vi "Main IU.vi"() -> ()   [LabVIEW 2018]
uses:
  <vilib>/Analysis/baseanly.llb/Mean (DBL).vi
  <vilib>/Analysis/NI_AALBase.lvlib
panel:
  out "Motor2":waveform(dbl)[](graph)
  out "Motor2":cluster{dbl, dbl, dbl}(graph)
  in  "Setpoint 2":dbl min=0.0 max=1.0 step=0.1
  out "rad/s":dbl(graph)
  out "Saving Data":bool
  in  "Record Button":bool
  in  "Filename":path=path "test.lvm"
  out "Motor1":waveform(dbl)[](graph)
  in  "Stop UI and RT":bool
  in  "Stop UI":bool
  in  "Setpoint1":dbl min=0.0 max=1.0 step=0.1
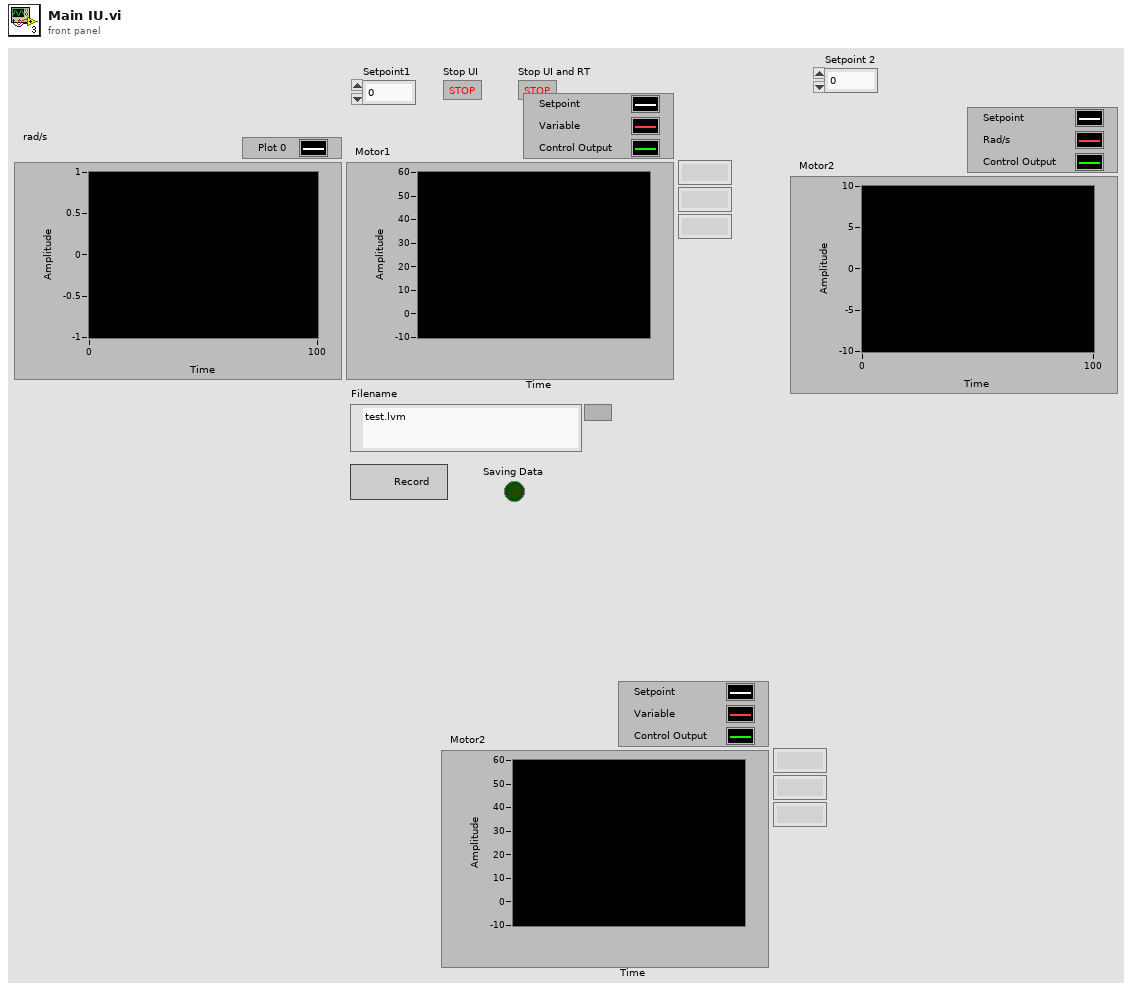
[diagram p1: front panel]
types:
  T1 = cluster{"Double":dbl, "dbl Scaled Value":dbl, "Output":dbl, "seconds since 1Jan1904":timestamp, dbl, dbl, dbl}
  T2 = cluster{"writer name":string, "Variant":variant, "Variant":variant}
  T3 = cluster{"Double":dbl, "dbl Scaled Value":dbl, "Output":dbl, "seconds since 1Jan1904":timestamp, dbl, dbl, dbl}[]
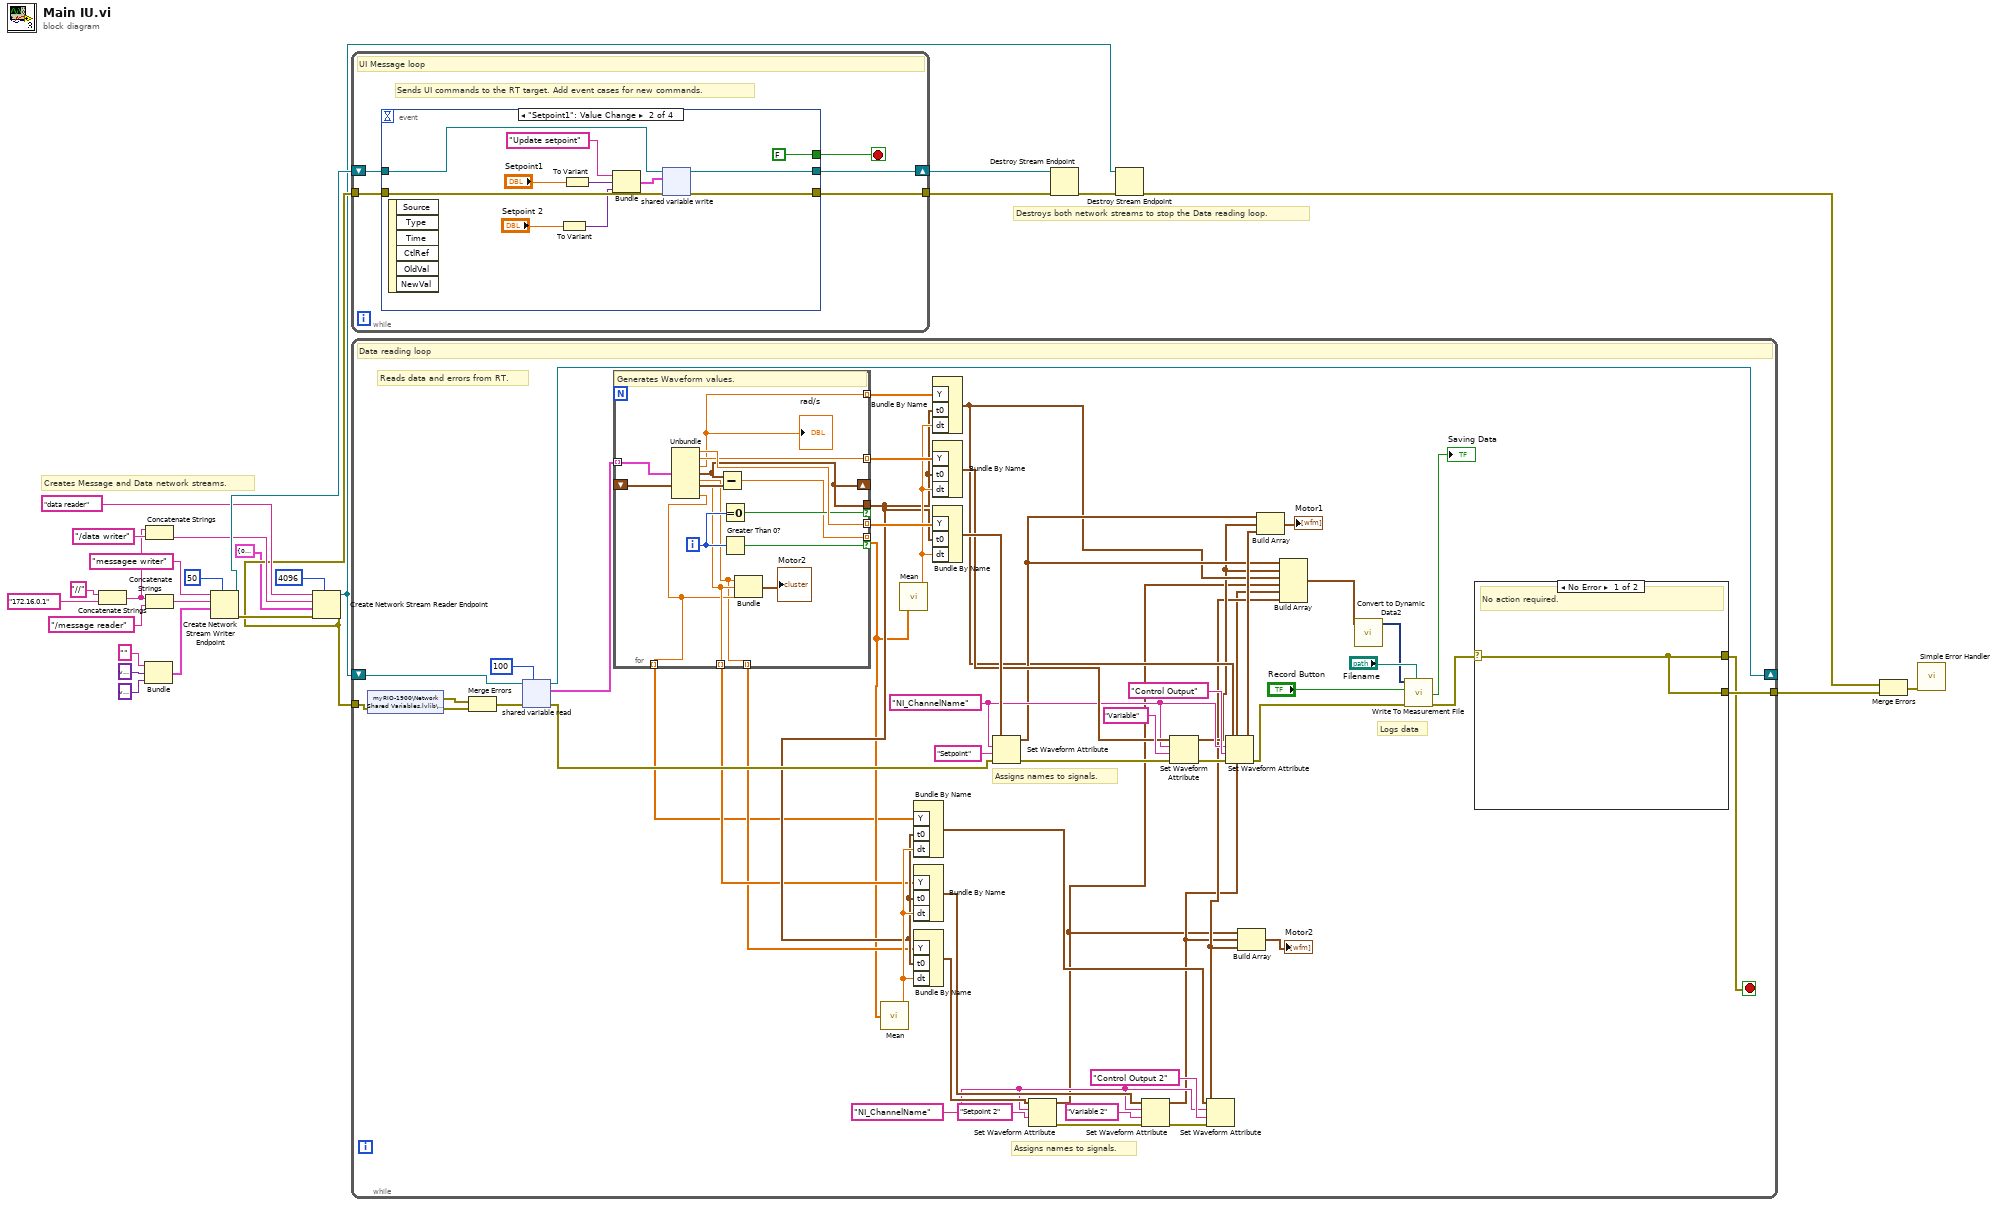
[diagram p0: block diagram]
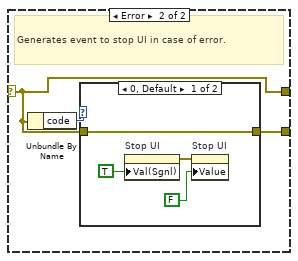
[diagram p2: hidden frame]
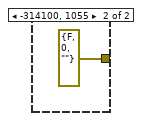
[diagram p3: hidden frame]
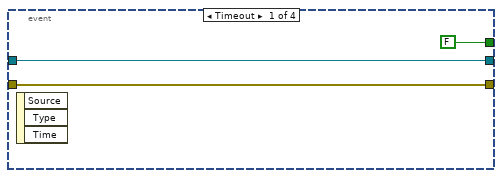
[diagram p4: hidden frame]
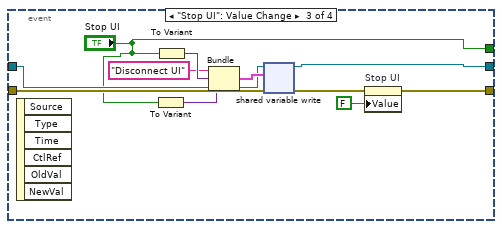
[diagram p5: hidden frame]
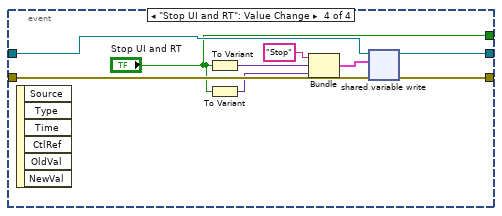
[diagram p6: hidden frame]
diagram:
  # "Destroys both network streams to stop the Data reading loop."
  # "Creates Message and Data network streams."
  n1 = Concatenate Strings("//", "172.16.0.1" ("myRIO IP")) -> (w2:string)
  n2 = Bundle("", variant, variant) -> (w26:cluster{string, variant, variant})  [unwired: 1 in]
  n3 = Concatenate Strings(w2, "/data writer") -> (w17:string)
  n4 = Concatenate Strings(w2, "/message reader") -> (w3:string)
  n5 = Create Network Stream Writer Endpoint(7:50 ("writer buffer size"), 9:w26, 10:w3, 11:"messagee writer" ("writer name")) -> (0:w14:errorcluster, 3:w20:refnum<k21>)  [unwired: 3 in]
  n6 = Create Network Stream Reader Endpoint(7:4096 ("reader buffer size"), 8:w14, 9:T1 {"Double"=0.0, "dbl Scaled Value"=0.0, "Output"=0.0, "seconds since 1Jan1904"=timestamp(0 s since 1904-01-01), 0.0, 0.0, 0.0} ("Data"), 10:w17, 11:"data reader" ("reader name")) -> (0:w13:errorcluster, 3:w6:refnum<k21>)  [unwired: 2 in]
  n7 = while {
    tunnel: w13 -> [w30]
    shift-right: [w29] -> w8
    shift-left: w20 -> [w31]
    tunnel: [w28] -> w9
    stop <- w27 stop-if-true
    # "Sends UI commands to the RT target. Add event cases for new commands."
    # "UI Message loop"
    n8 = event shown="[1] \"Setpoint1\": Value Change" {
      selector: _ -> [_ _ _ _]
      dyn-events: _ -> [_ _ _ _]
      timeout: _ -> [_ _ _ _]
      tunnel: w31 -> [w34 w45 w53 w59]
      tunnel: w30 -> [w32 w44 w50 w62]
      tunnel: [w34 w39 w52 w60] -> w29
      tunnel: [w32 w38 w48 w61] -> w28
      tunnel: [FALSE ("Stop UI and RT") FALSE ("Stop UI and RT") "Stop UI" "Stop UI and RT"] -> w27
      event Timeout {
        n9 = event-data() -> ()  [unwired: 1 in, 3 out]
      }
      event "Setpoint1": Value Change {
        n10 = event-data() -> ()  [unwired: 1 in, 6 out]
        n11 = To Variant(anything="Setpoint 2") -> (Variant=w35:variant)
        n12 = To Variant(anything="Setpoint1") -> (Variant=w43:variant)
        n13 = Bundle("writer name"="Update setpoint", "Variant"=w43, "Variant"=w35) -> (w40:T2)  [unwired: 1 in]
        n14 = shared-variable-write(w45, w44, w40) -> (w39:refnum<k21>, w38:errorcluster)  [unwired: 1 in, 1 out]
      }
      event "Stop UI": Value Change {
        n15 = event-data() -> ()  [unwired: 1 in, 6 out]
        n16 = To Variant(anything="Stop UI") -> (Variant=w47:variant)
        n17 = To Variant(anything="Stop UI") -> (Variant=w56:variant)
        n18 = Bundle("writer name"="Disconnect UI", "Variant"=w56, "Variant"=w47) -> (w55:T2)  [unwired: 1 in]
        n19 = shared-variable-write(w53, w50, w55) -> (w52:refnum<k21>, w49:errorcluster)  [unwired: 1 in, 1 out]
        n20 = property on="Stop UI" class="Bool (strict)"(error in=w49, "Value"=FALSE ("Stop UI and RT")) -> (error out=w48:errorcluster)  [unwired: 1 in, 1 out]
      }
      event "Stop UI and RT": Value Change {
        n21 = event-data() -> ()  [unwired: 1 in, 6 out]
        n22 = To Variant(anything="Stop UI and RT") -> (Variant=w65:variant)
        n23 = To Variant(anything="Stop UI and RT") -> (Variant=w58:variant)
        n24 = Bundle("writer name"="Stop", "Variant"=w65, "Variant"=w58) -> (w64:T2)  [unwired: 1 in]
        n25 = shared-variable-write(w59, w62, w64) -> (w60:refnum<k21>, w61:errorcluster)  [unwired: 1 in, 1 out]
      }
    }
  }
  n26 = while {
    tunnel: w13 -> [w94]
    shift-right: [w104] -> _
    shift-left: w6 -> [w119]
    tunnel: [w93] -> w10
    stop <- w92 stop-if-true
    w81 = "NI_ChannelName" ("name")
    w98 = "NI_ChannelName" ("name")
    # "Assigns names to signals."
    # "Logs data"
    # "Assigns names to signals."
    # "Reads data and errors from RT."
    # "Data reading loop"
    n27 = shared-variable "myRIO-1900\\Network Shared Variables.lvlib\\error IO"(error in=w94) -> (w97:errorcluster, error out=w96:errorcluster)
    n28 = Merge Errors(w97, w96) -> (w95:errorcluster)
    n29 = shared-variable-read(w119, w95, 100 ("# elements")) -> (w104:refnum<k21>, w109:errorcluster, w117:T3)  [unwired: 1 in, 1 out]
    n30 = for {
      tunnel: w117 -> [w142] mode=indexing
      tunnel: [w141] -> w116 mode=indexing
      tunnel: [w140] -> w115 mode=indexing
      tunnel: [w139] -> w91 mode=indexing
      tunnel: [w137] -> w80 if=w138
      shift-right: [w137] -> _
      shift-left: _ -> [w136]
      tunnel: [w135] -> w77 mode=indexing if=w133
      tunnel: [w130] -> w76 mode=indexing
      tunnel: [w131] -> w79 mode=indexing
      tunnel: [w129] -> w78 mode=indexing
      i -> [w134]
      # "Generates Waveform values."
      n31 = Unbundle(w142) -> ("Double"=w141:dbl, "dbl Scaled Value"=w140:dbl, "Output"=w139:dbl, "seconds since 1Jan1904"=w137:timestamp, w129:dbl, w131:dbl, w130:dbl)
      "rad/s" <- w139
      n32 = Subtract(x=w137, y=w136) -> (x-y=w135:dbl)
      n33 = Equal To 0?(x=w134) -> (x = 0?=w138:bool)
      n34 = Greater Than 0?(x=w134) -> (x > 0?=w133:bool)
      n35 = Bundle(w129, w131, w130) -> (→"Motor2":cluster{dbl, dbl, dbl})  [unwired: 1 in]
    }
    n36 = call-poly <vilib>:"Mean.vi"("X"=w77) -> ("mean"=w90:dbl)  [unwired: 1 out]
    n37 = call-poly <vilib>:"Mean.vi"("X"=w77) -> ("mean"=w114:dbl)  [unwired: 1 out]
    n38 = Bundle By Name("Y"=w76, "t0"=w80, "dt"=w90) -> (w82:waveform(dbl))  [unwired: 1 in]
    n39 = Bundle By Name("Y"=w79, "t0"=w80, "dt"=w90) -> (w83:waveform(dbl))  [unwired: 1 in]
    n40 = Bundle By Name("Y"=w78, "t0"=w80, "dt"=w90) -> (w89:waveform(dbl))  [unwired: 1 in]
    n41 = Bundle By Name("Y"=w91, "t0"=w80, "dt"=w114) -> (w71:waveform(dbl))  [unwired: 1 in]
    n42 = Bundle By Name("Y"=w115, "t0"=w80, "dt"=w114) -> (w106:waveform(dbl))  [unwired: 1 in]
    n43 = Bundle By Name("Y"=w116, "t0"=w80, "dt"=w114) -> (w113:waveform(dbl))  [unwired: 1 in]
    n44 = Set Waveform Attribute(4:w109, 5:"Setpoint" ("name"), 6:w98, 7:w113) -> (0:w108:errorcluster, 3:w72:waveform(dbl))  [unwired: 1 out]
    n45 = Set Waveform Attribute(5:"Setpoint 2" ("name"), 6:w81, 7:w89) -> (0:w85:errorcluster, 3:w67:waveform(dbl))  [unwired: 1 in, 1 out]
    n46 = Set Waveform Attribute(4:w85, 5:"Variable 2" ("name"), 6:w81, 7:w83) -> (0:w84:errorcluster, 3:w68:waveform(dbl))  [unwired: 1 out]
    n47 = Set Waveform Attribute(4:w108, 5:"Variable" ("name"), 6:w98, 7:w106) -> (0:w107:errorcluster, 3:w70:waveform(dbl))  [unwired: 1 out]
    n48 = Set Waveform Attribute(4:w84, 5:"Control Output 2" ("name"), 6:w81, 7:w82) -> (3:w69:waveform(dbl))  [unwired: 2 out]
    n49 = Set Waveform Attribute(4:w107, 5:"Control Output" ("name"), 6:w98, 7:w71) -> (0:w103:errorcluster, 3:w105:waveform(dbl))  [unwired: 1 out]
    n50 = Build Array(w67, w68, w69) -> (→"Motor2":waveform(dbl)[])
    n51 = Build Array(w72, w70, w105) -> (→"Motor1":waveform(dbl)[])
    n52 = Build Array(w72, w70, w71, w67, w68, w69) -> (w66:waveform(dbl)[])
    n53 = call "Convert to Dynamic Data2"("Array of Waveforms"=w66) -> ("Dynamic Data Type"=w74:dynamicdata)  [unwired: 3 in]
    n54 = call "Write To Measurement File"("Signals"=w74, "Enable"="Record Button", "error in (no error)"=w103, "Filename"="Filename") -> ("Saving Data"=→"Saving Data":bool, "error out"=w99:errorcluster)  [unwired: 13 in, 1 out]
    n55 = case shown="No Error" w99 {
      selector: w99 -> [w120 w121]
      tunnel: [w120 w122] -> w93
      tunnel: [w120 w121] -> w92
      frame No Error {
        # "No action required."
      }
      frame Error {
        # "Generates event to stop UI in case of error."
        n56 = Unbundle By Name(w121) -> ("code"=w123:i32)
        n57 = case shown="0, Default" w123 {
          tunnel: [w126 errorcluster {"status"=FALSE, "code"=0, "source"=""} ("error IO")] -> w122
          tunnel: w121 -> [w126 _]
          frame 0, Default {
            n58 = property on="Stop UI" class="Bool (strict)"("Val(Sgnl)"=TRUE ("Stop UI and RT")) -> (error out=w125:errorcluster)  [unwired: 2 in, 1 out]
            n59 = property on="Stop UI" class="Bool (strict)"(error in=w125, "Value"=FALSE ("Stop UI")) -> ()  [unwired: 1 in, 2 out]
          }
          frame -314100, 1055 {
          }
        }
      }
    }
  }
  n60 = Destroy Stream Endpoint(8:w9, 11:w8) -> (0:w7:errorcluster)
  n61 = Destroy Stream Endpoint(8:w7, 11:w6) -> (0:w5:errorcluster)
  n62 = Merge Errors(w5, w10) -> (w11:errorcluster)
  n63 = call <vilib>:"Simple Error Handler.vi"("error in (no error)"=w11) -> ()  [unwired: 4 in, 5 out]
